vi "Open Error Codes List.vi"(6 "Variant in":variant, 7 "Shift Pressed?":bool, 8 "error in (no error)":errorcluster, 10 "QD Combo Box Ref":refnum<vi>, 11 "QD Launch VI Ref":refnum<vi>) -> (0 "error out":errorcluster, 4 "Variant out":variant)   [LabVIEW 2017]
doc: "Opens error codes list window and enables to insert codes on the block diagram.\n\nDefault Shortcut - [L]"
uses:
  UI/Controls/Error Codes List Window States.ctl
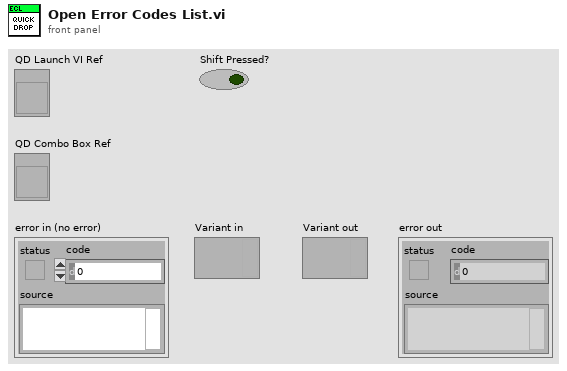
[diagram p1: front panel]
types:
  T1 = typedef "Error Codes List Window States.ctl" = enum16{"init", "load project errors", "parse combo box", "update list view", "open FP", "close", "idle", "add error", "remove error", "edit error", "edit file", "change scope", "filter"}
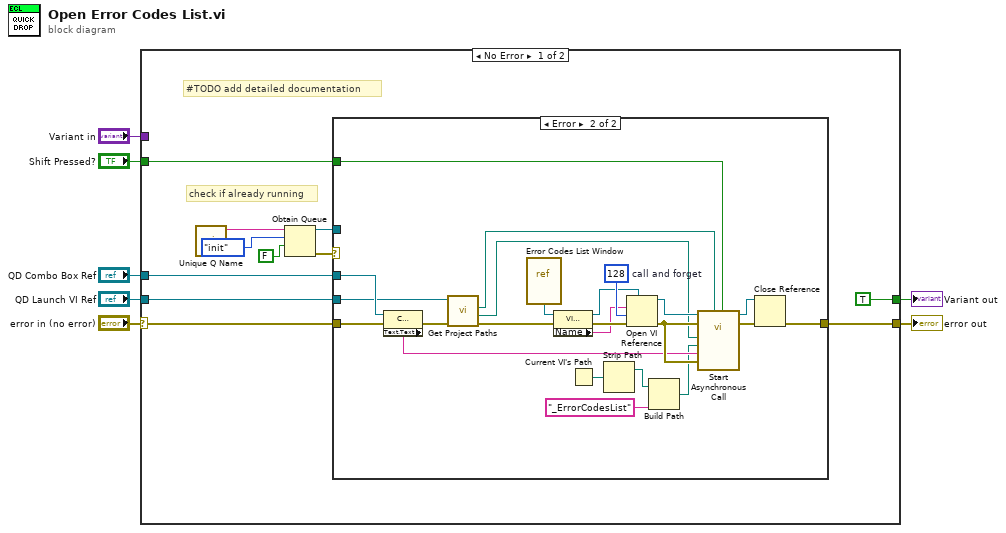
[diagram p0: block diagram]
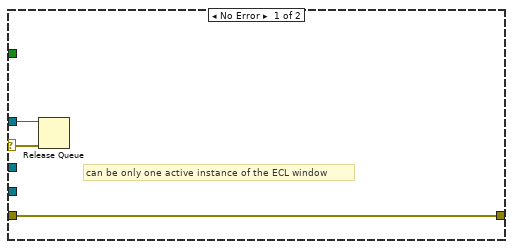
[diagram p2: hidden frame]
diagram:
  n1 = case shown="No Error" "error in (no error)" {
    selector: "error in (no error)" -> [w14 w45]
    tunnel: [w16 w45] -> w3
    tunnel: "QD Launch VI Ref" -> [w15 _]
    tunnel: "Shift Pressed?" -> [w8 _]
    tunnel: "QD Combo Box Ref" -> [w17 _]
    tunnel: [TRUE _] -> w2
    tunnel: "Variant in" -> [_ _]
    frame No Error {
      # "#TODO add detailed documentation"
      # "check if already running"
      n2 = call "Unique Q Name.vi"() -> ("unique Q name"=w10:string)  [unwired: 11 in]
      n3 = Obtain Queue(name (unnamed)=w10, element data type=Error_Codes_List_Window_States."init" ("states"), create if not found? (T)=FALSE) -> (queue out=w11:refnum<queue>, error out=w12:errorcluster)  [unwired: 2 in, 1 out]
      n4 = case shown="Error" w12 {
        selector: w12 -> [w19 _]
        tunnel: w17 -> [_ w40]
        tunnel: [w21 w28] -> w16
        tunnel: w15 -> [_ w33]
        tunnel: w14 -> [w21 w31]
        tunnel: w11 -> [w20 _]
        tunnel: w8 -> [_ w25]
        frame No Error {
          # "can be only one active instance of the ECL window"
          n5 = Release Queue(queue=w20, error in (no error)=w19) -> ()  [unwired: 1 in, 3 out]
        }
        frame Error {
          w43 = 128  # call and forget
          n6 = property class="CmbBox"(reference=w40, error in=w31) -> (error out=w30:errorcluster, "Text.Text"=w29:string)  [unwired: 1 out]
          n7 = call "Get Project Paths.vi"("error in (no error)"=w30, "VI in"=w33) -> ("error out"=w32:errorcluster, "project errors path"=w23:path, "project path"=w22:path)  [unwired: 6 in, 1 out]
          n8 = vi-ref "Error Codes List Window.vi"() -> (w34:refnum<vi>)
          n9 = property class="VI (strict)"(reference=w34, error in=w32) -> (reference out=w26:refnum<vi>, error out=w44:errorcluster, "Name"=w35:string)
          n10 = Current VI's Path() -> (path=w39:path)
          n11 = Strip Path(path=w39) -> (stripped path=w38:path)  [unwired: 1 out]
          n12 = Open VI Reference(type specifier VI Refnum (for type only)=w26, vi path=w35, options=w43, error in (no error)=w44) -> (vi reference=w42:refnum<vi>, error out=w41:errorcluster)  [unwired: 2 in]
          n13 = Build Path(base path=w38, name or relative path="_ErrorCodesList") -> (appended path=w24:path)
          n14 = call-by-ref "Start Asynchronous Call"(reference=w42, error in=w41, "shift pressed?"=w25, "project file"=w22, 8:"error in (no error)"=w41, "combo box text"=w29, "scripting templates directory"=w24, "project error file"=w23) -> (reference out=w27:refnum<vi>, error out=w36:errorcluster)  [unwired: 6 in]
          n15 = Close Reference(reference=w27, error in (no error)=w36) -> (error out=w28:errorcluster)
        }
      }
    }
    frame Error {
    }
  }
  "error out" <- w3
  "Variant out" <- w2
